vi "Handle path to driver DLL.vi"(8 "error in (no error)":errorcluster, 11 "Path to DLL":path=path "C:/Program Files (x86)/National Instruments/LabVIEW 2017/instr.lib/ANC350/Win64/anc350v4.dll") -> (0 "error out":errorcluster, 3 "path out":path=path "C:/Program Files (x86)/National Instruments/LabVIEW 2017/instr.lib/ANC350/Win64/anc350v4.dll")   [LabVIEW 2022 SP3, in "SampleRotator.lvlib"]
doc: "At first, verifies given path. If the path is incorrect, searches in library directory, and in \"LabVIEW/instr directory\". If cannot find the driver DLL, it will prompt an user.\n\ninputs: path.\n\nOutputs: path; error cluster."
uses:
  SampleRotator.lvlib
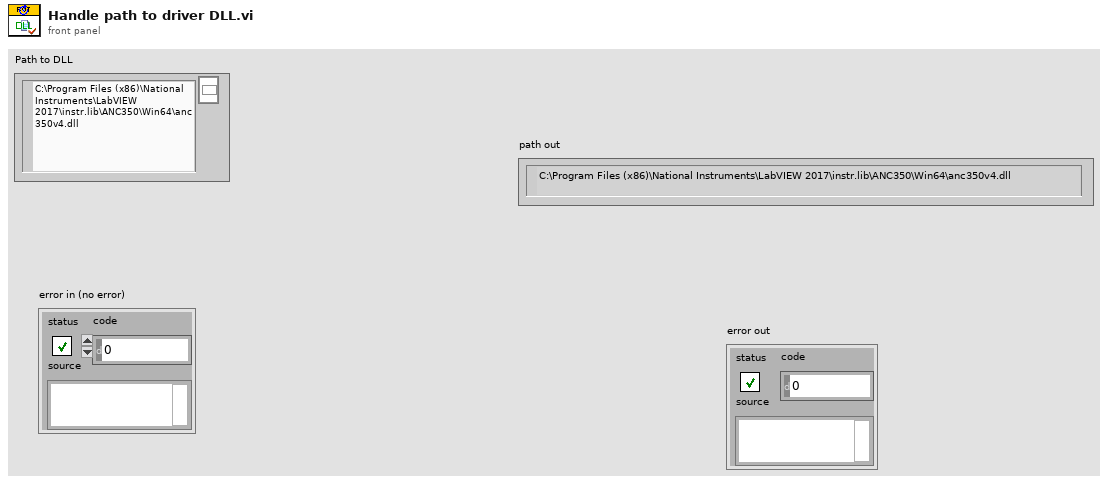
[diagram p1: front panel]
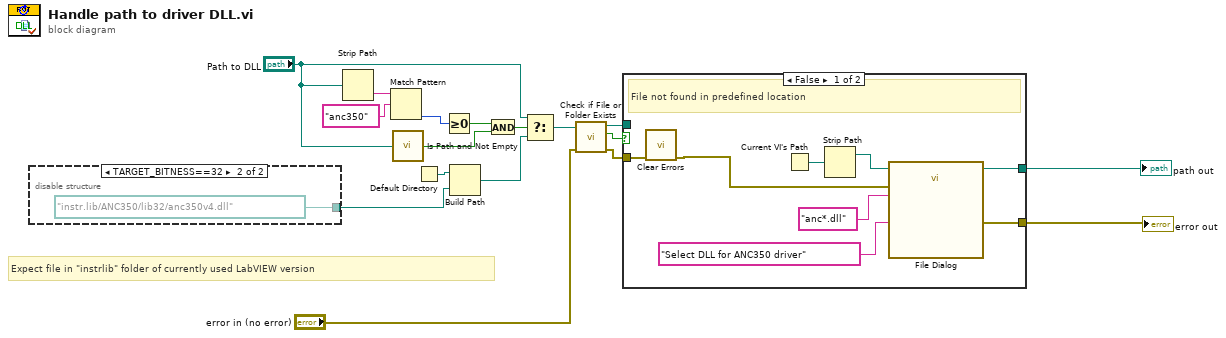
[diagram p0: block diagram]
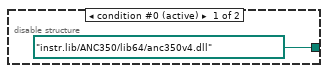
[diagram p2: hidden frame]
diagram:
  # "Expect file in \"instrlib\" folder of currently used LabVIEW version"
  n1 = disable-structure shown="TARGET_BITNESS==32" {
    disable-tunnel: [path "instr.lib/ANC350/lib64/anc350v4.dll" ("Path to *.DLL 2") path "instr.lib/ANC350/lib32/anc350v4.dll" ("Path to *.DLL 2")] -> w2
    frame condition #0 (active) {
    }
    frame condition #1 {
    }
  }
  n2 = Strip Path(path="Path to DLL") -> (name=w11:string)  [unwired: 1 out]
  n3 = Match Pattern(string=w11, regular expression="anc350" ("pattern (all files)")) -> (offset past match=w9:i32)  [unwired: 1 in, 3 out]
  n4 = call <vilib>:"Is Path and Not Empty.vi"("path"="Path to DLL") -> ("Is Path and Not Empty?"=w5:bool)  [unwired: 4 in]
  n5 = Default Directory() -> (w4:path)
  n6 = Greater Or Equal To 0?(x=w9) -> (x >= 0?=w7:bool)
  n7 = Build Path(base path=w4, name or relative path=w2) -> (appended path=w3:path)
  n8 = And(x=w7, y=w5) -> (x .and. y?=w8:bool)
  n9 = Select(t="Path to DLL", s=w8, f=w3) -> (s? t:f=w14:path)
  n10 = call <vilib>:"Check if File or Folder Exists.vi"("error in (no error)"="error in (no error)", "path"=w14) -> ("error out"=w15:errorcluster, "file or folder exists?"=w13:bool, "dup path"=w12:path)  [unwired: 7 in]
  n11 = case shown="False" w13 {
    tunnel: w12 -> [_ w29]
    tunnel: [w27 w29] -> w17
    tunnel: [w26 w28] -> w16
    tunnel: w15 -> [w25 w28]
    frame False {
      # "File not found in predefined location"
      n12 = call <vilib>:"Clear Errors.vi"("error in (no error)"=w25) -> ("error out"=w20:errorcluster)  [unwired: 5 in, 1 out]
      n13 = Current VI's Path() -> (path=w22:path)
      n14 = Strip Path(path=w22) -> (stripped path=w21:path)  [unwired: 1 out]
      n15 = call "File Dialog"("start path"=w21, "prompt"="Select DLL for ANC350 driver", "error in"=w20, "pattern (all files)"="anc*.dll") -> ("selected path"=w27:path, "error out"=w26:errorcluster)  [unwired: 8 in, 2 out]
    }
    frame True {
    }
  }
  "path out" <- w17
  "error out" <- w16
